vi "LBCB Position DAO.vi"(0 "LBCB Settings Actions":T4, 3 "Config Ref Number":T3, 5 "LBCB Number":T1, 7 "LBCB Position In":T2={"Motion Center"=[0.0, 0.0, 0.0], "Transformation Matrix"=[[1.0, 0.0, 0.0, 0.0, 0.0, 0.0], [0.0, 1.0, 0.0, 0.0, 0.0, 0.0], [0.0, 0.0, 1.0, 0.0, 0.0, 0.0], [0.0, 0.0, 0.0, 1.0, 0.0, 0.0], [0.0, 0.0, 0.0, 0.0, 1.0, 0.0], [0.0, 0.0, 0.0, 0.0, 0.0, 1.0]]}, 11 "error in (no error)":errorcluster) -> (8 "LBCB Position Output":T2={"Motion Center"=[0.0, 0.0, 0.0], "Transformation Matrix"=[[1.0, 0.0, 0.0, 0.0, 0.0, 0.0], [0.0, 1.0, 0.0, 0.0, 0.0, 0.0], [0.0, 0.0, 1.0, 0.0, 0.0, 0.0], [0.0, 0.0, 0.0, 1.0, 0.0, 0.0], [0.0, 0.0, 0.0, 0.0, 1.0, 0.0], [0.0, 0.0, 0.0, 0.0, 0.0, 1.0]]}, 14 "Config Ref Number out":T3, 15 "error out":errorcluster)   [LabVIEW 2013]
uses:
  Metadata/Persistant DAO Actions.ctl
  <vilib>/Utility/config.llb/Config Data RefNum.ctl
  Metadata/LBCB Position.ctl
  Metadata/LBCB Number.ctl
  <vilib>/Utility/config.llb/Write Key (Double).vi
  <vilib>/Utility/config.llb/Read Key (Double).vi
  <vilib>/Utility/config.llb/NI_LVConfig.lvlib
panel:
  in  "Keys":string[](array[string])=["Dx", "Dy", "Dz", "Rx", "Ry", "Rz"]
  # "Y"
  # "(inch)"
  # "XLBCB CMD = T-1*XLBCB OM"
  # "Z"
  # "(inch)"
  # "XOM DISP = T*XLBCB DISP"
  # "(inch)"
  # "Dx"
  # "Dy"
  # "Dz"
  # "Rx"
  # "Ry"
  # "Rz"
  # "Dx"
  # "Dy"
  # "Dz"
  # "Rx"
  # "Ry"
  # "Rz"
  # "Y"
  # "(inch)"
  # "XLBCB CMD = T-1*XLBCB OM"
  # "Z"
  # "(inch)"
  # "XOM DISP = T*XLBCB DISP"
  # "(inch)"
  # "Dx"
  # "Dy"
  # "Dz"
  # "Rx"
  # "Ry"
  # "Rz"
  # "Dx"
  # "Dy"
  # "Dz"
  # "Rx"
  # "Ry"
  # "Rz"
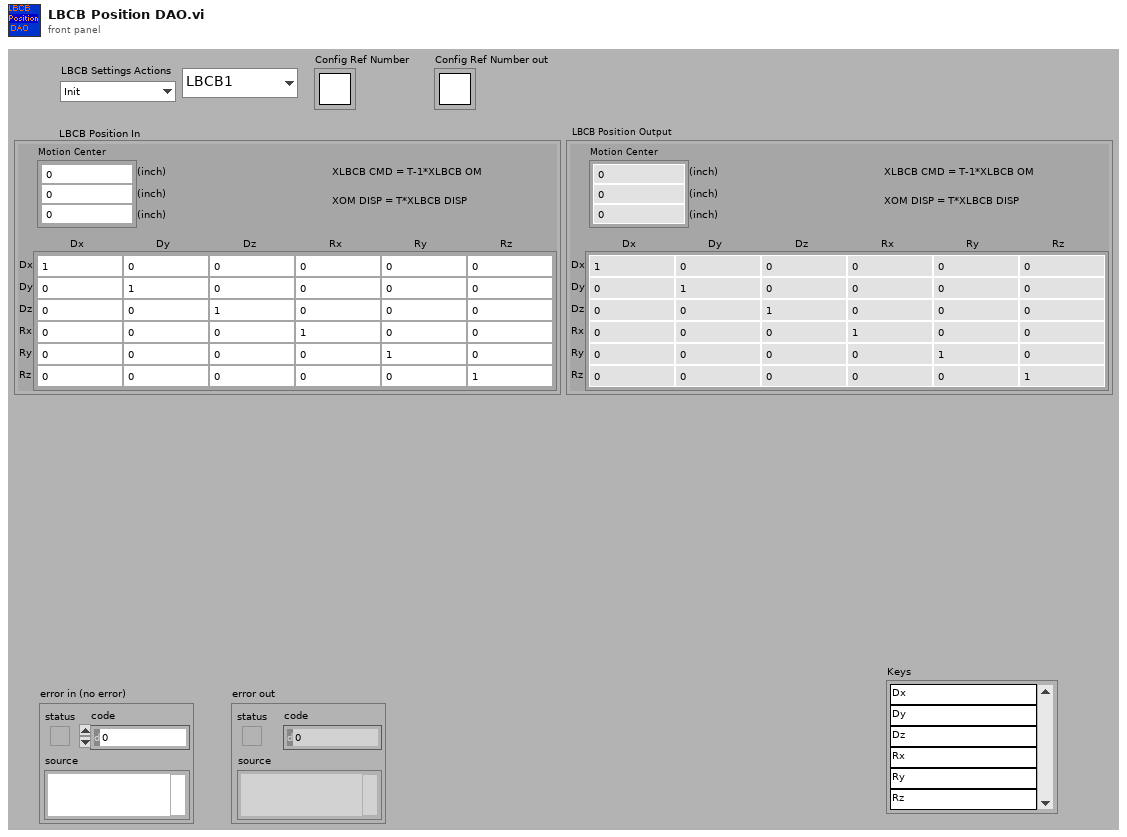
[diagram p1: front panel]
types:
  T1 = typedef "LBCB Number.ctl" = enum16{"LBCB1", "LBCB2"}
  T2 = typedef "LBCB Position.ctl" = cluster{"Motion Center":dbl[], "Transformation Matrix":dbl[][]}
  T3 = typedef "NI_LVConfig.lvlib/Config Data RefNum.ctl" = refnum<k1>
  T4 = typedef "Persistant DAO Actions.ctl" = enum16{"Init", "Get", "Set", "Load", "Save"}
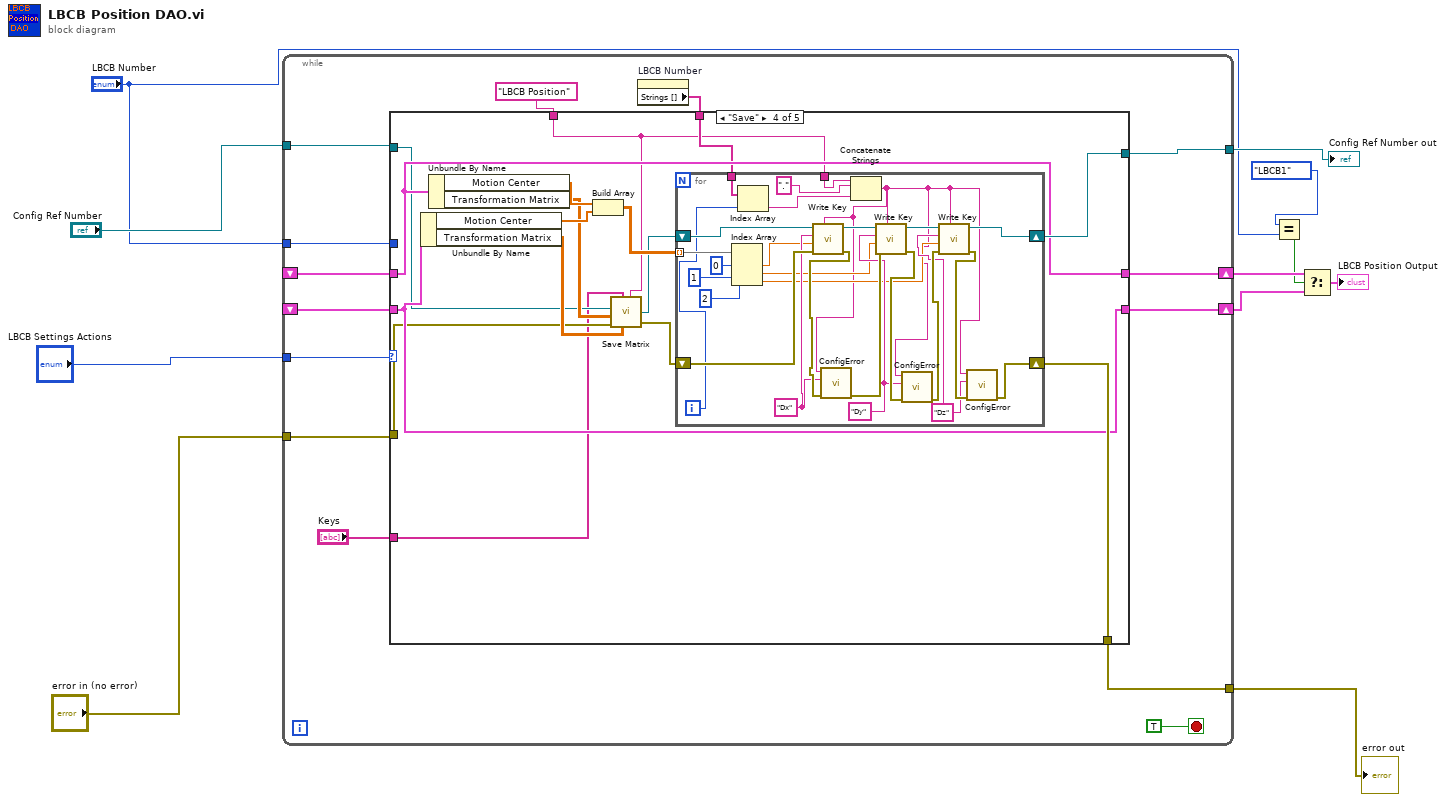
[diagram p0: block diagram]
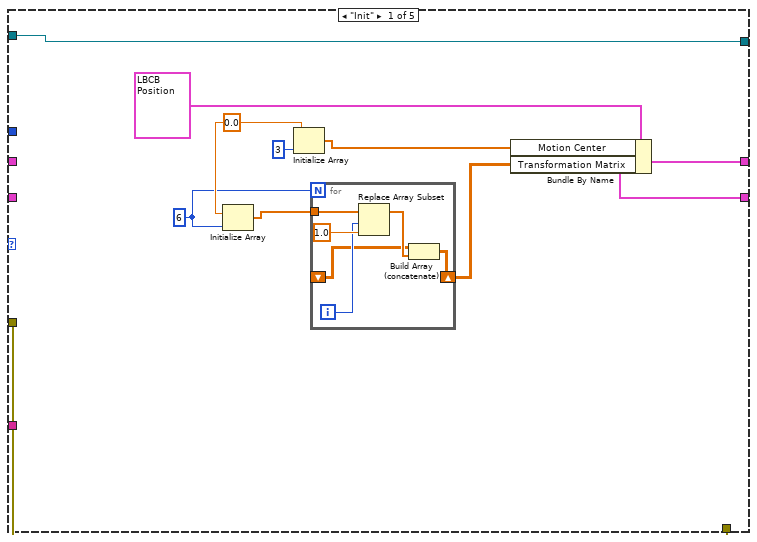
[diagram p2: hidden frame]
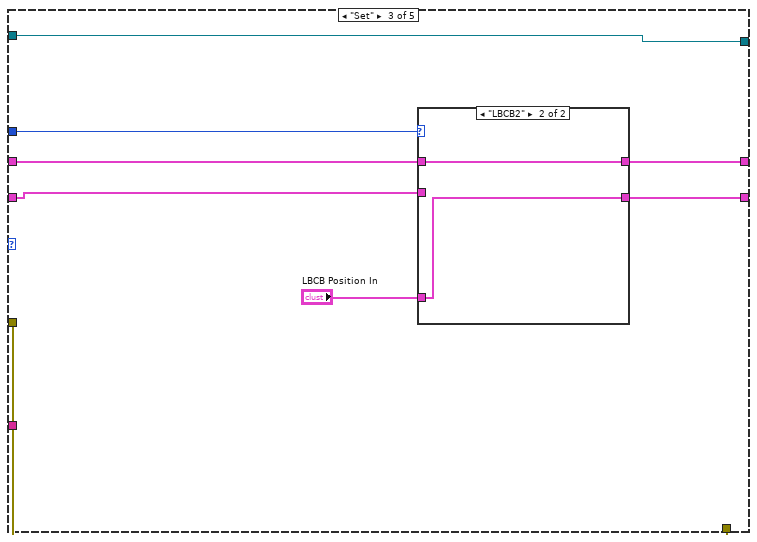
[diagram p4: hidden frame]
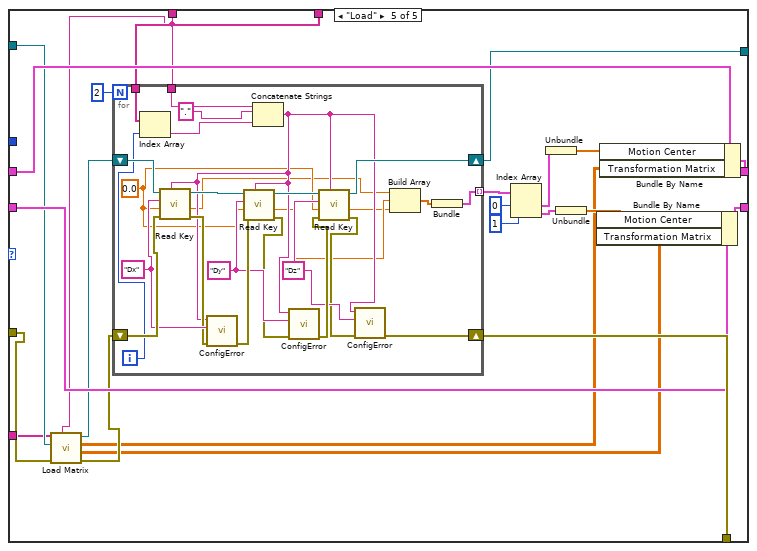
[diagram p6: hidden frame]
diagram:
  n1 = while {
    tunnel: "LBCB Settings Actions" -> [w24]
    tunnel: "Config Ref Number" -> [w23]
    tunnel: "error in (no error)" -> [w21]
    tunnel: [w20] -> w8
    tunnel: [w19] -> w7
    shift-right: [w18] -> w5
    shift-left: _ -> [w17]
    shift-right: [w16] -> w4
    shift-left: _ -> [w15]
    tunnel: "LBCB Number" -> [w14]
    stop <- TRUE stop-if-true
    n2 = property on="LBCB Number" class="Enum (strict)"() -> ("Strings []"=w13:string[])  [unwired: 2 in, 2 out]
    n3 = case shown="\"Save\"" w24 {
      tunnel: "LBCB Position" ("section") -> [_ _ _ w58 w107]
      tunnel: w23 -> [w34 w44 w52 w62 w106]
      tunnel: w21 -> [w35 w45 w53 w64 w109]
      tunnel: [w34 w44 w52 w73 w121] -> w20
      tunnel: [w35 w45 w53 w72 w120] -> w19
      tunnel: [w31 w43 w46 w71 w122] -> w18
      tunnel: w17 -> [_ w43 w50 w71 w123]
      tunnel: [w31 w42 w47 w70 w119] -> w16
      tunnel: w15 -> [_ w42 w49 w70 w118]
      tunnel: w14 -> [_ _ w51 _ _]
      tunnel: w13 -> [_ _ _ w60 w117]
      tunnel: "Keys" -> [_ _ _ w59 w102]
      frame "Init" {
        w29 = 0.0 ("element")
        w28 = 6 ("index")
        n4 = Initialize Array(w29, w28) -> (w27:dbl[])
        n5 = Initialize Array(w29, 3 ("dimension size")) -> (w30:dbl[])
        n6 = for {
          N: w28 -> [_]
          tunnel: w27 -> [w41]
          shift-right: [w40] -> w26
          shift-left: _ -> [w36]
          i -> [w38]
          n7 = Replace Array Subset(array=w41, new element=1.0 ("new element/subarray"), index=w38) -> (w37:dbl[])
          n8 = Build Array (concatenate)(w36, w37) -> (w40:dbl[][])
        }
        n9 = Bundle By Name(cluster=T2 {"Motion Center"=[0.0, 0.0, 0.0], "Transformation Matrix"=[[1.0, 0.0, 0.0, 0.0, 0.0, 0.0], [0.0, 1.0, 0.0, 0.0, 0.0, 0.0], [0.0, 0.0, 1.0, 0.0, 0.0, 0.0], [0.0, 0.0, 0.0, 1.0, 0.0, 0.0], [0.0, 0.0, 0.0, 0.0, 1.0, 0.0], [0.0, 0.0, 0.0, 0.0, 0.0, 1.0]]} ("LBCB Settings Output"), "Motion Center"=w30, "Transformation Matrix"=w26) -> (w31:T2)
      }
      frame "Get" {
      }
      frame "Set" {
        n10 = case shown="\"LBCB2\"" w51 {
          tunnel: w50 -> [_ w57]
          tunnel: w49 -> [w55 _]
          tunnel: "LBCB Position In" -> [w54 w56]
          tunnel: [w55 w56] -> w47
          tunnel: [w54 w57] -> w46
          frame "LBCB1" {
          }
          frame "LBCB2" {
          }
        }
      }
      frame "Save" {
        n11 = Unbundle By Name(w70) -> ("Motion Center"=w68:dbl[], "Transformation Matrix"=w65:dbl[][])
        n12 = Unbundle By Name(w71) -> ("Motion Center"=w69:dbl[], "Transformation Matrix"=w66:dbl[][])
        n13 = Build Array(w69, w68) -> (w67:dbl[][])
        n14 = call "Save Matrix.vi"("section"=w58, "Matrix 2"=w65, "error in (no error)"=w64, "Matrix 1"=w66, "Keys"=w59, "refnum in"=w62) -> ("error out"=w63:errorcluster, "refnum out"=w61:T3)  [unwired: 3 out]
        n15 = for {
          tunnel: w58 -> [w88]
          shift-right: [w87] -> w73
          shift-left: w61 -> [w99]
          shift-right: [w86] -> w72
          shift-left: w63 -> [w100]
          tunnel: w67 -> [w85] mode=indexing
          tunnel: w60 -> [w78]
          i -> [w77]
          w89 = "Dz" ("key")
          w90 = "Dy" ("key")
          w91 = "Dx" ("key")
          n16 = Index Array(array=w85, index #1=0 ("index"), index #2=1 ("index"), index #3=2 ("index")) -> (element #1=w81:dbl, element #2=w80:dbl, element #3=w79:dbl)
          n17 = Index Array(array=w78, index=w77) -> (element=w74:string)
          n18 = Concatenate Strings(w88, "." ("string"), w74) -> (w76:string)
          n19 = call-poly <vilib>:"Write Key.vi"("section"=w76, "error in (no error)"=w100, "value"=w81, "key"=w91, "refnum"=w99) -> ("error out"=w96:errorcluster, "refnum out"=w98:T3)  [unwired: 3 in, 2 out]
          n20 = call "ConfigError.vi"("error in (no error)"=w96, "Key"=w91, "Section"=w76) -> ("error out"=w95:errorcluster)  [unwired: 8 out]
          n21 = call-poly <vilib>:"Write Key.vi"("section"=w76, "error in (no error)"=w95, "value"=w80, "key"=w90, "refnum"=w98) -> ("error out"=w94:errorcluster, "refnum out"=w97:T3)  [unwired: 3 in, 2 out]
          n22 = call "ConfigError.vi"("error in (no error)"=w94, "Key"=w90, "Section"=w76) -> ("error out"=w93:errorcluster)  [unwired: 8 out]
          n23 = call-poly <vilib>:"Write Key.vi"("section"=w76, "error in (no error)"=w93, "value"=w79, "key"=w89, "refnum"=w97) -> ("error out"=w92:errorcluster, "refnum out"=w87:T3)  [unwired: 3 in, 2 out]
          n24 = call "ConfigError.vi"("error in (no error)"=w92, "Key"=w89, "Section"=w76) -> ("error out"=w86:errorcluster)  [unwired: 8 out]
        }
      }
      frame "Load" {
        n25 = call "Load Matrix.vi"("section"=w107, "error in (no error) 2"=w109, "refnum in"=w106, "Keys"=w102) -> ("error in (no error)"=w108:errorcluster, "Matrix 2"=w103:dbl[][], "Matrix 1"=w104:dbl[][], "refnum out"=w105:T3)  [unwired: 4 out]
        n26 = for {
          N: 2 -> [_]
          tunnel: w107 -> [w131]
          shift-right: [w137] -> w121
          shift-left: w105 -> [w148]
          shift-right: [w136] -> w120
          shift-left: w108 -> [w149]
          tunnel: w117 -> [w132]
          tunnel: [w124] -> w116 mode=indexing
          i -> [w133]
          w129 = 0.0
          w139 = "Dz" ("key")
          w142 = "Dy" ("key")
          w145 = "Dx" ("key")
          n27 = Index Array(array=w132, index=w133) -> (element=w135:string)
          n28 = Concatenate Strings(w131, "." ("string"), w135) -> (w130:string)
          n29 = call-poly <vilib>:"Read Key.vi"("section"=w130, "error in (no error)"=w149, "default value"=w129, "key"=w145, "refnum"=w148) -> ("error out"=w144:errorcluster, "value"=w128:dbl, "refnum out"=w147:T3)  [unwired: 4 out]
          n30 = call "ConfigError.vi"("error in (no error)"=w144, "Key"=w145, "Section"=w130) -> ("error out"=w143:errorcluster)  [unwired: 8 out]
          n31 = call-poly <vilib>:"Read Key.vi"("section"=w130, "error in (no error)"=w143, "default value"=w129, "key"=w142, "refnum"=w147) -> ("error out"=w141:errorcluster, "value"=w127:dbl, "refnum out"=w146:T3)  [unwired: 4 out]
          n32 = call "ConfigError.vi"("error in (no error)"=w141, "Key"=w142, "Section"=w130) -> ("error out"=w140:errorcluster)  [unwired: 8 out]
          n33 = call-poly <vilib>:"Read Key.vi"("section"=w130, "error in (no error)"=w140, "default value"=w129, "key"=w139, "refnum"=w146) -> ("error out"=w138:errorcluster, "value"=w126:dbl, "refnum out"=w137:T3)  [unwired: 4 out]
          n34 = call "ConfigError.vi"("error in (no error)"=w138, "Key"=w139, "Section"=w130) -> ("error out"=w136:errorcluster)  [unwired: 8 out]
          n35 = Build Array(w128, w127, w126) -> (w125:dbl[])
          n36 = Bundle(w125) -> (w124:cluster{dbl[]})  [unwired: 1 in]
        }
        n37 = Index Array(array=w116, index #1=0 ("index"), index #2=1 ("index")) -> (element #1=w113:cluster{dbl[]}, element #2=w111:cluster{dbl[]})
        n38 = Unbundle(w113) -> (w112:dbl[])
        n39 = Unbundle(w111) -> (w110:dbl[])
        n40 = Bundle By Name(cluster=w118, "Motion Center"=w110, "Transformation Matrix"=w103) -> (w119:T2)
        n41 = Bundle By Name(cluster=w123, "Motion Center"=w112, "Transformation Matrix"=w104) -> (w122:T2)
      }
    }
  }
  "error out" <- w7
  "Config Ref Number out" <- w8
  n42 = Equal?(x=LBCB_Number."LBCB1", y="LBCB Number") -> (x = y?=w3:bool)
  n43 = Select(t=w5, s=w3, f=w4) -> (s? t:f=→"LBCB Position Output":T2)
